vi "Get Results Indexes.vi"(11 "data dictionary in":refnum<class "data dictionary.lvclass">) -> (0 "error out":errorcluster, 2 "Results Indexes":T1)   [LabVIEW 2015, in "Sequencer Module tests.lvlib"]
uses:
  Sequencer Module tests.lvlib
  <vilib>/NI/Tag Bus/dictionary/data dictionary.lvclass
  Results Indexes.ctl
  <vilib>/NI/Tag Bus/dictionary/data dictionary.lvclass/data dictionary.ctl
  <vilib>/NI/Tag Bus/dictionary/lookup polymorphs/locate Boolean.vi
  <vilib>/NI/Tag Bus/dictionary/lookup polymorphs/locate I32.vi
  <vilib>/NI/Tag Bus/dictionary/search/find data index.vi
  <vilib>/NI/Tag Bus/dictionary/search/search string list.vi
  <vilib>/NI/Tag Bus/dictionary/tag not found.vi
panel:
  in  "error in (no error)":errorcluster
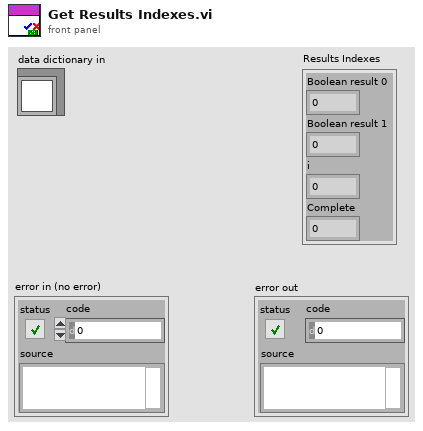
[diagram p1: front panel]
types:
  T1 = typedef "Sequencer Module tests.lvlib/Results Indexes.ctl" = cluster{"Boolean result 0":i32, "Boolean result 1":i32, "i":i32, "Complete":i32}
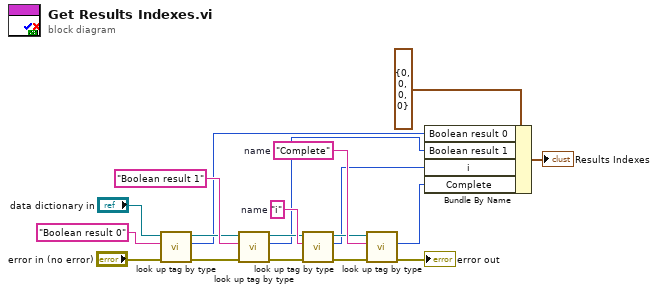
[diagram p0: block diagram]
diagram:
  w14 = "i"  # name
  w15 = "Complete"  # name
  n1 = call-poly <vilib>:"look up tag by type.vi"("error in"="error in (no error)", "name"="Boolean result 0", "data dictionary in"="data dictionary in") -> ("error out"=w16:errorcluster, "index"=w4:i32, "data dictionary out"=w10:refnum<class "data dictionary.lvclass">)  [unwired: 6 in]
  n2 = call-poly <vilib>:"look up tag by type.vi"("error in"=w16, "name"="Boolean result 1", "data dictionary in"=w10) -> ("error out"=w17:errorcluster, "index"=w3:i32, "data dictionary out"=w12:refnum<class "data dictionary.lvclass">)  [unwired: 6 in]
  n3 = call-poly <vilib>:"look up tag by type.vi"("error in"=w17, "name"=w14, "data dictionary in"=w12) -> ("error out"=w18:errorcluster, "index"=w2:i32, "data dictionary out"=w13:refnum<class "data dictionary.lvclass">)  [unwired: 6 in]
  n4 = call-poly <vilib>:"look up tag by type.vi"("error in"=w18, "name"=w15, "data dictionary in"=w13) -> ("error out"=→"error out":errorcluster, "index"=w1:i32)  [unwired: 6 in, 1 out]
  n5 = Bundle By Name(cluster=T1 {"Boolean result 0"=0, "Boolean result 1"=0, "i"=0, "Complete"=0} ("Results Indexes"), "Boolean result 0"=w4, "Boolean result 1"=w3, "i"=w2, "Complete"=w1) -> (→"Results Indexes":T1)
